vi "Window_Processing.vi"(11 "Array in":dbl[][](array[numeric])) -> (3 "Array out":sgl[](array[numeric]))   [LabVIEW 2020]
uses:
  <vilib>/Analysis/baseanly.llb/Mean (DBL).vi
  <vilib>/Analysis/NI_AALBase.lvlib
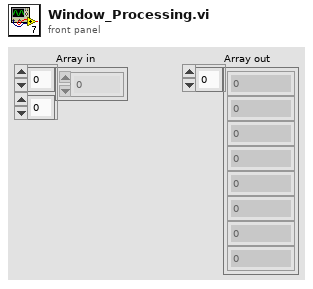
[diagram p1: front panel]
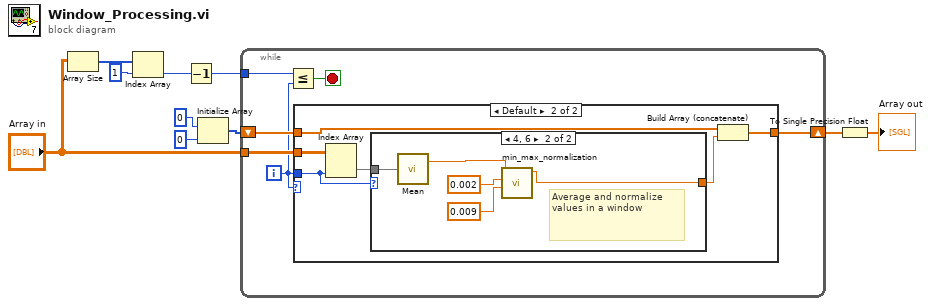
[diagram p0: block diagram]
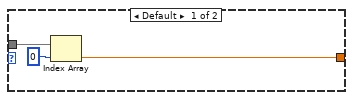
[diagram p3: hidden frame]
diagram:
  n1 = Array Size(array="Array in") -> (size(s)=w2:i32[])
  n2 = Index Array(array=w2, index=1) -> (element=w7:i32)
  n3 = Decrement(x=w7) -> (x-1=w8:i32)
  n4 = Initialize Array(0, 0) -> (w6:i32[])
  n5 = while {
    tunnel: "Array in" -> [w16]
    tunnel: w8 -> [w15]
    shift-right: [w11] -> w9
    shift-left: w6 -> [w13]
    i -> [w12]
    stop <- w14 stop-if-true
    n6 = Less Or Equal?(x=w15, y=w12) -> (x <= y?=w14:bool)
    n7 = case shown="Default" w12 {
      tunnel: w16 -> [_ w23]
      tunnel: w12 -> [_ w21]
      tunnel: w13 -> [w17 w22]
      tunnel: [w17 w20] -> w11
      frame 3, 5, 7 {
      }
      frame Default {
        n8 = Index Array(array=w23, index (col)=w21) -> (element=w19:dbl[])  [unwired: 1 in]
        n9 = case shown="4, 6" w21 {
          tunnel: [w24 w29] -> w18
          tunnel: w19 -> [w25 w28]
          frame Default {
            n10 = Index Array(array=w25, index=0) -> (element=w24:dbl)
          }
          frame 4, 6 {
            # "Average and normalize values in a window"
            n11 = call-poly <vilib>:"Mean.vi"("X"=w28) -> ("mean"=w27:dbl)  [unwired: 1 out]
            n12 = call "min_max_normalization.vi"("Numeric 3"=0.009, "Numeric in"=0.002, "mean"=w27) -> ("Numeric out"=w29:dbl)  [unwired: 8 in]
          }
        }
        n13 = Build Array (concatenate)(w22, w18) -> (w20:dbl[])
      }
    }
  }
  n14 = To Single Precision Float(number=w9) -> (single precision float=→"Array out":sgl[])
